vi "Status Monitor Port Number--Const.vi"() -> (3 "Status Monitor Port":i32)   [LabVIEW 2017, in "Communications Library.lvlib"]
doc: "Port where status messages are made available."
uses:
  Communications Library.lvlib
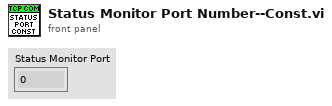
[diagram p1: front panel]
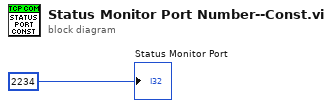
[diagram p0: block diagram]
diagram:
  "Status Monitor Port" <- 2234 ("timeout ms (default 25000ms)")
